vi "Configure Channel.vi"(8 "error in":errorcluster, 10 "Settings":T1 {"Fall Time" format="%#_g s"; "Rise Time" format="%#_g s"; "Pulse Width" format="%#_g s"; "Symmetry" format="%#_g %"; "Phase" format="%#_g °"; "Offset" format="%#_g V"; "Amplitude" format="%#_g V"; "Frequency" format="%#_g Hz"}, 11 "336XX in":refnum<class "336XX.lvclass">) -> (0 "error out":errorcluster, 3 "336XX out":refnum<class "336XX.lvclass">)   [LabVIEW 2019, in "336XX.lvlib" / "336XX.lvclass"]
uses:
  Library/336XX.lvclass
  C:/Users/Public/Documents/Development/builds/Instruments/FunctionGenerator.lvlibp/Library/FunctionGenerator.lvclass
  builds/Instruments/FunctionGenerator.lvlibp/Custom Controls/WaveformSettings.ctl
  builds/Instruments/FunctionGenerator.lvlibp/Custom Controls/WaveformMode.ctl
  builds/Instruments/FunctionGenerator.lvlibp/Accessors/Read Active Channel.vi
  builds/Instruments/FunctionGenerator.lvlibp/Library/FunctionGenerator.lvclass
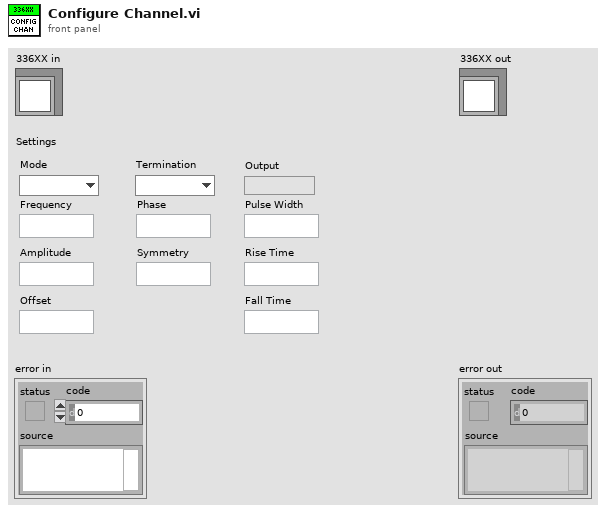
[diagram p1: front panel]
types:
  T1 = typedef "FunctionGenerator.lvlibp/FunctionGenerator.lvclass/WaveformSettings.ctl" = cluster{"Frequency":dbl, "Amplitude":dbl, "Offset":dbl, "Phase":dbl, "Symmetry":dbl, "Pulse Width":dbl, "Rise Time":dbl, "Fall Time":dbl, "Mode":T2, "Termination":enum16{"50_Ohm", "High_Z"}, "Output":bool}
  T2 = typedef "FunctionGenerator.lvlibp/FunctionGenerator.lvclass/WaveformMode.ctl" = enum16{"Sine", "Square", "Ramp", "Pulse", "Arbitrary", "Triangle", "Noise", "DC"}
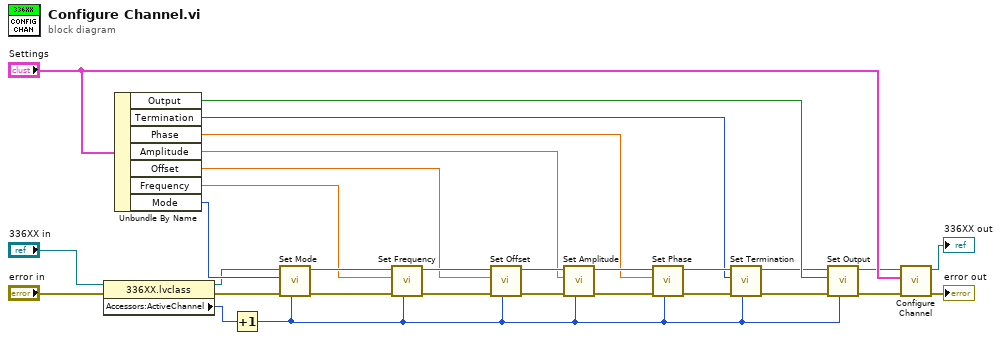
[diagram p0: block diagram]
diagram:
  n1 = property class="336XX.lvclass"(reference="336XX in", error in="error in") -> (reference out=w3:refnum<class "336XX.lvclass">, error out=w5:errorcluster, "Accessors:ActiveChannel"=w2:i32)
  n2 = Unbundle By Name("Settings") -> ("Output"=w11:bool, "Termination"=w6:enum16{"50_Ohm", "High_Z"}, "Phase"=w14:dbl, "Amplitude"=w17:dbl, "Offset"=w20:dbl, "Frequency"=w24:dbl, "Mode"=w27:T2)
  n3 = Increment(x=w2) -> (x+1=w1:i32)
  n4 = call "Set Mode.vi"("Channel"=w1, "error in (no error)"=w5, "Waveform"=w27, "336XX in"=w3) -> ("error out"=w25:errorcluster, "336XX out"=w26:refnum<class "336XX.lvclass">)  [unwired: 6 in]
  n5 = call "Set Frequency.vi"("Channel"=w1, "error in (no error)"=w25, "Frequency"=w24, "336XX in"=w26) -> ("error out"=w21:errorcluster, "336XX out"=w22:refnum<class "336XX.lvclass">)  [unwired: 6 in]
  n6 = call "Set Offset.vi"("Channel"=w1, "error in (no error)"=w21, "Offset"=w20, "336XX in"=w22) -> ("error out"=w19:errorcluster, "336XX out"=w18:refnum<class "336XX.lvclass">)  [unwired: 6 in]
  n7 = call "Set Amplitude.vi"("Channel"=w1, "error in (no error)"=w19, "Amplitude"=w17, "336XX in"=w18) -> ("error out"=w15:errorcluster, "336XX out"=w16:refnum<class "336XX.lvclass">)  [unwired: 6 in]
  n8 = call "Set Phase.vi"("Channel"=w1, "error in (no error)"=w15, "phase"=w14, "336XX in"=w16) -> ("error out"=w9:errorcluster, "336XX out"=w10:refnum<class "336XX.lvclass">)  [unwired: 6 in]
  n9 = call "Set Termination.vi"("Channel"=w1, "error in (no error)"=w9, "Termination"=w6, "336XX in"=w10) -> ("error out"=w8:errorcluster, "336XX out"=w7:refnum<class "336XX.lvclass">)  [unwired: 6 in]
  n10 = call "Set Output.vi"("Channel"=w1, "error in (no error)"=w8, "Output"=w11, "336XX in"=w7) -> ("error out"=w12:errorcluster, "336XX out"=w13:refnum<class "336XX.lvclass">)  [unwired: 6 in]
  n11 = call-parent "Configure Channel.vi"("error in (no error)"=w12, "Settings"="Settings", "FunctionGenerator in"=w13) -> ("error out"=→"error out":errorcluster, "FunctionGenerator out"=→"336XX out":refnum<class "336XX.lvclass">)  [unwired: 7 in]
